vi "Main_12a.vi"() -> ()   [LabVIEW 2023]
uses:
  ENUM_Type.ctl
  <vilib>/Utility/error.llb/Trim Whitespace One-Sided.vi
panel:
  out "Complete Match Count":i32
  out "Answer":i32
  in  "Puzzle":string="??#.????#???.#?# 1,5,1,1,1\n?##?##??#? 7,1\n??????#???. 1,7\n??#?#??#.?#.??#? 5,1,1,2\n???????.??? 1,3\n?#..##?##??###??#? 2,13\n?.????????.???????? 1,5,1,6\n?.???#???. 2,2\n??#..#???#? 1,1,4\n?.?##?????#??? 1,5,2,1\n.???#?????##??#.? 3,8\n?????????????.#.. 4,3,1\n..#???????.? 4,3,1\n????#??.?.#??? 7,3\n#??#???##??.?? 4,1,3,2\n??#?#?##?.???#??. 6,5\n???.#??.??###?.#?? 3,1,5,2\n?.????##??#?? 6,3\n???..?##????.? 2,3,1\n?.?#????.??#?#.? 1,2,1,3,1\n?.?###.???? 4,2\n?#???..??##? 4,3\n???#????#?. 1,2,3\n#???#???#??#???.? 1,10,1\n???????????????????? 1,5,6,3\n???????#??? 2,6\n??.??.????.?#?????# 1,1,2,1,4,3\n???#???.??#? 1,4,1,1\n???#???##??##? 3,2,3\n????.??????#?.#? 1,1,1,4,2\n?.#??#???? 1,1,5\n??##???#?.##??..? 4,2,4\n??????#.????.# 4,2,1,1\n??????#??#?.??? 2,7,1\n.????????##.?.?.##? 5,2,1,1,2\n.??????????#?#. 3,1,2,1\n?????????????. 2,1,5\n?##????#?.?????.#??? 2,1,2,3,3\n?????????#?.?????#? 1,2,1,3,4,2\n..?.#???.?##.? 1,3,2\n.??????????????? 10,2\n?.?#????#?.??? 1,1,2,2\n??????.#??.?.? 1,1,1\n#???#?#??#????? 1,2,1,5\n???.?.??#????.? 3,6\n.#.???###???.#?..??? 1,8,2,2\n.???.??#????# 2,4,1\n.????#?#?? 3,3,1\n?###??#??## 4,2,2\n??#?#???#???.??. 3,5,1\n???####??##..?#.#.?? 9,2,1,1\n??#?#???#.?. 5,1\n???#????#???##?# 2,3,3,1\n?#???????#???#??? 1,3,3,3,1\n#???#????#.##..? 8,1,2\n?????.?#?#??? 1,5\n.??#.??#?.? 1,1,1\n?#?#???#???.??? 1,1,4,1,3\n.????#.?.#??? 1,1,2,1\n.??#?.??#? 4,2\n#????????. 1,4,1\n??.#?#????#?...?? 1,8,2\n?#.#?#.??##? 2,3,1,2\n...??.?#?? 1,1\n?.?.????#..? 1,2,1\n?##????????.??.?#??? 6,1,1,4\n?.??#.??.?.???? 3,2\n.????.?????.???.?? 4,1,1,3,1\n?????????##???????#? 2,1,1,2,2,2\n???.?????.????? 2,3,5\n???#??????.??#??.? 1,6,1,1,1\n??##??????###??? 12,1\n?.??.?????? 1,1,2\n??#??????#?.. 2,5\n???#####????. 1,8\n.?#?##??????#??.???? 6,2,1\n?.#??#???????#????? 1,1,12,1\n??????????#.?..?##? 1,1,1,1,3,3\n???????#???.??## 10,4\n.?#????.?.???..? 1,1,2\n.???#?#????? 2,2,1\n#????#?.????##?#?# 1,5,1,5,1\n???.##??????##??#? 1,2,8,2\n??#????????????#? 6,7\n????.??.#.?#?#? 1,1,1,1,4\n??##?#??.#???? 6,1,4\n?#?.?#????????#?. 3,2,4,3\n..??????##?# 2,1,2,1\n?????????.???? 4,1,1,1\n.??#?????.?.?. 1,6,1\n#.?#?#??????#??# 1,6,2,1,1\n.#?.#.##??# 1,1,5\n??#?????#?????? 5,4\n.#??.?.?.? 2,1\n.?#???##.????##?? 7,2\n?#?.??????#??????# 1,8,3\n?.#??#??.?#.. 4,1,1\n?#?#?#??????? 7,1,1\n?#???????? 6,1\n????#..?#???##? 1,1,2,3\n..?????#?###??.? 1,9,1\n?##???.???#?# 4,4\n??.??#???..??#? 1,2,1,3\n#?#??????.??#?? 8,1,3\n???#?##?#?? 2,6\n.?.???#???.#?????? 1,3,1,5,1\n?#.???????# 2,2,1\n?.???.??.? 1,1,1\n?#?#?#??????#??#??? 1,5,2,4,2\n?#??.?#?????.?#. 4,6,2\n#???.?#?#??#?.??#? 2,7,1\n.??#...???????. 3,1,1\n?..???##??. 1,6\n??#??#?#??? 2,4\n?.?.??.??????#?. 1,7\n?.?????????.??. 2,2,2\n???.?????? 2,1\n???.??????????? 1,3,4,1\n?#????#???#??? 10,1\n??#???.?????#???# 6,3,1\n????.?##??#??# 3,8\n?????????????. 1,7,1\n?..?????.#???.. 1,4,2\n?.???#???#? 1,5,1\n#???.????? 2,1,1\n?#.??#?.???? 1,1,1,1\n????.?#???.???. 1,1,4,2\n.?#??#??.??????? 2,4,6\n.??.?##.??#?#.??? 2,3,2,1,1\n..??????#?.?? 2,2\n???#?#??.##. 3,2,2\n?..?????????##?#??? 1,13,1\n??#?????#?.??#?????? 6,2,5,2\n???.???#???# 1,1,3,1\n??##????.?. 4,1\n??#??#??#?. 3,6\n.??????#????#.#.?? 1,1,8,1,1\n?#?#?.?.?.###??#???? 5,1,1,3,1,1\n???.#?#???.?? 1,1,5,1\n?????####??????? 2,5,2,1\n????.??#??#? 1,1,2,1\n??.?????#?#.????? 2,3,3\n?#??#?#?.????.??? 2,3,2,2\n?????????#??.??????. 1,6,1,1,1,1\n???.##?##??#? 1,6,1\n????#?.??.. 4,1\n?#??#?#???.????#?# 4,4,6\n?????#??#.#? 1,2,2,1\n?#?#?#??###??? 1,1,7\n.##?.????? 3,3\n??#???###????? 1,6\n.?###????????##?#?? 7,1,5\n..?#????????#? 3,5\n#?#???.??? 1,1,1\n#???????????#??.??? 10,3,1\n???##??#??#?.?????. 10,3\n?#?????.???????## 3,2,5,3\n??.??#####???. 2,8\n???.?????? 1,1,3\n???#???????????. 6,4\n#???#?????##???.?#? 2,1,1,5,2\n?#?..???#??????. 2,7,2\n?????##?#? 2,3,2\n.#?..????# 2,3\n???????#??#.?..??.. 3,1,1,2,1,1\n?.#??#????? 1,3,2\n???..?.?.? 1,1,1\n?#.?#??#???.##.? 1,1,4,2\n???#?#.??#??? 4,1\n??????#????.???? 6,1,1,1,2\n???..??.#???? 1,1,1,2\n????????.? 1,1,1\n?..#??.??. 3,1\n?##.??#??? 2,1,1\n?????#?????#?#?? 2,12\n?#??????#???.?? 1,6,2,1\n#??.???.??##???.#? 2,3,7,2\n???????..????#????? 2,1,1,7,1\n????#??.?????? 1,2,4\n?###?#?##?##??.??. 12,1\n?#??#.?.??#?... 3,1,1,1,2\n??#??#??#????#? 9,2\n???????##????? 1,1,5\n?.?#????#?.??.?? 3,3,1,1\n???..??????#..??#? 1,1,7,1,1\n??.???###???#..? 1,1,5,1,1\n??.??.#????#????# 2,1,7,2\n??????#?#??????# 1,6,1\n#?.?...??.??????? 1,1,1,6\n??#?##??#?..## 7,2\n?#?###..?.#?##??.?.# 5,6,1\n.??.?.???. 2,1,1\n?.???..?.?#?.??.???? 1,3\n.#?.??????.?.?#??? 2,6,4\n???##...??. 3,1\n????????????#?????. 4,6\n????#.??#? 1,1,1\n?.?#.??..??#?????..? 1,2,1,8\n?????.??.? 1,2,1\n??????##?.?? 1,4\n???.????#??? 1,1,5\n.??#???.#.#??#??. 6,1,2,1,1\n?.????#??##?????? 1,1,1,7\n??????##.??? 3,2,1\n?.????#?????.?.? 1,4,2,1\n?????????????## 1,1,2,4\n.?##??#??.??# 4,1,3\n??#?##??#?? 2,5,1\n?????.###??.?.#??# 1,1,4,1,1,1\n.????????##?#? 1,7\n??????????.? 7,1\n.?????###????..#. 12,1\n????.????? 3,1,1\n#.??#????#????#????? 1,5,1,7,1\n.##??????.??##? 7,3\n?..?.???#?????###? 1,1,5,5\n??????#???. 1,1,3\n??.#???????##????. 1,2,3,6\n?.?.?.?.#???????#?. 1,1,1,1,2,7\n?????#????????. 1,1,1,4,1\n?.??#??#?? 1,1,2\n??#???.#.?#?#?? 1,1,1,1,5\n?????????.? 4,1\n??.?????#?.?.#?? 7,1\n??.?#.?????#??. 2,7\n?????##..? 1,4\n?????????. 4,1\n??.?..?#???? 2,3,2\n????.####??###? 2,4,4\n?####???##??????? 10,1,1\n???#?#???# 1,5,1\n????###.??.?????#??. 6,1,6\n#???????#?. 2,1,4\n?#?.???##???????#? 3,1,2,1,6\n???#??#?.?.?????? 1,5,1,1,4\n?.#???##???.?.## 1,3,2,2\n???..##?.?.? 2,2,1\n?.#?#?????. 3,1\n????.##?#?#??##?? 3,12\n#?##???????? 1,3,3,1\n???.#?.????##? 1,2,1,4\n???.??#???? 1,3\n.???###??.???????# 7,5,1\n?#.??.?#???##?. 1,1,1,4\n.????###????? 2,6\n???#???.???????#?? 1,2,1,3,4,1\n.?.?????????? 3,5\n??#???#?.###????.?? 7,3,1,1,1\n#??###??#?#.????? 11,1\n#.?????#??#.##???.? 1,1,7,5\n??????.????#???? 1,1,4,1,1\n?.?#?#?#??###?? 7,4\n????#???#?#?###????? 1,2,10,1\n????#????? 1,4,2\n???.#??#????.?#??.?. 3,2,1,1,4,1\n?????.?#??????. 1,2,1,1,1\n?#???????#?#?#???.? 2,12\n?#??..??.???###?? 4,2,1,5\n##????????#.? 5,2\n#?#?.?.??###??#?. 4,8\n??##?.???? 3,4\n?.????##???????? 8,1,1\n#????#??#???#?#.??? 15,1\n?.?????.#? 4,2\n?.##???..?? 1,3,1\n#????#??????????#?? 2,7,2,3\n???.????#? 1,1,2\n??..#?????### 1,3\n????????.?? 2,4,1\n#??##??#.?????.??? 1,5,2,1,1,1\n???#.?#?#?. 3,1,2\n?##?#??????#?#.# 3,3,3,1,1\n??.#?..??? 1,1,1\n?#??.???#? 1,1,3\n???#???????.??##?? 8,3\n??.#.?#???#??.? 2,1,7\n??????.####?.?#?# 4,4,4\n??????????? 2,2,1\n?#?.??.???.? 2,2\n????#?#?## 6,2\n.??###??????.? 5,3\n.???#.#????? 3,5\n?##?#?.?#?#??. 6,2,1,1\n#.???.??#?####?..? 1,1,1,8,1\n????#???#???# 1,1,2,3\n?????.??.#???#? 3,5\n?#??..?????????#?. 1,1,3,1,4\n#?????????????.?? 6,1,1,1\n?#?????..?????#??# 3,1,1,5\n???????.???????????? 1,4,1,9\n.????????????.. 2,1,6\n.?#??????. 2,4\n??#??#???#.???#? 1,5,2,1,2\n.?.???????.?.#??? 4,1,2\n##?.??##?..???. 3,4,3\n??..??#??#?. 1,6\n??#??????????##???? 2,6,4,1\n??..????##?????? 1,5\n##????????.??.#??? 2,6,4\n?#??#...?????# 2,2,1,2\n?..??????.???.?# 1,1,3,1,1\n.?###??#???#???? 7,4,1\n?#?.?????. 2,2\n??..????.?????# 1,1,2,2\n??##.#??????.##??#?? 1,2,1,1,1,5\n??.##??????#???#??? 4,8\n??#?????????. 4,3,2\n#????.???? 1,1,1\n?..??.?????? 2,3\n??????#??###???? 1,1,9,1\n?????#?#???????.. 1,6,3\n?#??.???#?##. 3,3,2\n?..##?#???????#?? 9,1\n???.?#?#?#?. 1,5\n???##?#???#?# 8,3\n?##??#??.??.???????? 2,3,1,6\n.??...?????????#.#? 1,6,2,2\n????.#??#?#.##?. 1,1,1,3,3\n?#?#?????.??????. 5,3\n??.????##???. 1,5\n????#?.???? 2,1\n????..??#???. 4,2,1\n???????.?# 2,1\n????????????? 1,1,3\n???##??????###.?#? 2,2,2,3,1\n??????#?#?#?#?## 3,10\n?????#??..????????? 8,5\n??##???????.??? 6,1,1,2\n?.???.????.??? 3,1,1,3\n.?.???.??? 1,2\n.???###???#??.?? 5,1,1,1\n????#?.##?###.# 1,3,2,3,1\n.?#???????? 1,4\n?#?#?????????### 8,6\n?????..???.???? 4,3,1,1\n..?#?.?#??? 1,5\n.????.??#? 3,3\n?##????.?#??????..?? 7,3,3,1\n?????##??.?.??...?? 9,2,2\n??..#??####??.?.?#? 8,2\n??????##????? 1,1,6\n??????#??.???#? 7,5\n???#..??.????. 4,1,2\n.#?.?###??? 1,4\n????###?...?#?#? 8,4\n?????#???#??????? 1,1,6,1,1\n.??#?#?##??????? 7,1,1\n.#.?????#.?#### 1,2,1,1,5\n?#??..#??.#?? 3,1,1,1\n????#??.???. 3,1,3\n#.???#???. 1,2\n???.???##.???.? 1,1,2,2\n?#?#..?#????##?.?. 3,9\n.?.??.????? 2,2\n??????.?.##?#?.? 5,4\n???#???.????? 7,1\n??####?????.???#?? 6,3,4\n?.?...?#.#?#??? 1,2,5\n??.??#??#?#?#??.?? 2,3,7,1\n?#?.???????? 1,1,1\n????????#?##?#??? 1,2,9,1\n#???.???#????.??#??? 3,1,1,1,4,1\n.??#?.?.#??? 2,1,2,1\n.?##?###.###?#?.??. 6,5,2\n.?.???????#????##? 3,10\n?.##???..#? 5,2\n????????????#??.???? 1,1,10,1\n??##??#.??#??#?? 5,3,2,1\n?#???#.??????..# 6,4,1,1\n????????.? 1,2,2\n?????#??#??#????#??? 14,2,1\n???#??.???#?#???? 4,7,1\n.?.##?.???#??..????? 1,3,4,2\n??????#??????? 1,1\n..#?##??.????. 5,3\n??????????#.? 4,1\n#????.???.? 1,1\n.?..?#.??? 2,1\n?#.??##??.##?.?? 2,4,2,2\n??#????#??????? 9,1\n.#?.##?##.#???? 1,5,1,1\n?#?###???#??#?.??? 11,1,1\n???#??..?? 3,1\n#?#??????#?????#? 12,2\n??#?#?.???.? 2,2,3,1\n?#???.?.??#?#???? 5,1,8\n.???#?#??#?????. 10,1\n??????.?????.? 5,1,1,1\n.?.??????????# 3,7\n.#?.??..##??.?#..#? 1,1,4,2,1\n?##?#??.??###?????# 2,1,1,1,7,1\n?##?.???.? 2,1,1\n?????#.#?##.?#? 1,1,4,1\n?#?.??.?#.#.##.? 2,1,1,1,2\n???????.#.??##??.?. 6,1,3,1,1\n.?#??#???????#???.#. 3,1,1,2,4,1\n?????#?.##??##??.?? 1,2,2,3,2\n#??.???????? 1,1,1,1\n????#?.##?.?#?#?# 5,2,5\n.?.??.#?????????..?# 1,1,6,1,2\n???#?#?????. 7,2\n???????##??#?.?#?.? 1,8,3\n.?..?#?#???? 4,1\n??.?#??.????. 1,1,3\n????##???##???#??? 12,4\n?###?#??..#?.??? 6,1,2,1\n##??..##?#????# 3,2,1,1\n?????#?##??##???#?? 2,13\n#?..???##???##?#???? 2,6,4,1,1\n.????.?....#????. 1,3\n?.?.??#??#.?# 1,2,1,2\n???#??.??#.? 1,1,1,2\n.????#?#???#??????? 12,1,1\n?..#??#?##??#???? 1,1,2,3,5\n.#??##?##??????.?# 2,11,2\n.?.#?#?.?#???#.? 1,4,6\n?#.##??.????? 2,4,4\n???.??????.??. 2,1,1,2\n???????.?##.#???.? 1,1,1,2,3,1\n??..???????#?.? 5,2\n?????#????? 3,2,2\n.##????..#??.. 6,2\n????.??????.???###? 3,3,1,5\n??????#?.???# 1,3,1,1\n????#????. 6,1\n??.?#????. 1,4\n??????#???##???. 6,1,3,1\n?.?#.????. 1,1,4\n?##??.#?#??.#?? 3,1,1,1,1\n?.?#??????. 1,5,1\n???????#?. 1,4\n???#????#?##?#?????? 2,2,1,1,6,1\n??##.?????##??#.? 1,2,7,1\n????????.# 4,1\n.???#????? 1,1,1\n?.?#??.????.?#?? 1,4,2,2,1\n.?##?#???.??..?#? 3,3,3\n?#??.?.?#??? 1,1,4\n????..#????#.?? 1,1,1,3,2\n???#?..??? 5,1\n?##???##.?. 3,2,1\n??#???.???### 2,1,1,3\n????.?#??##?. 2,2,2\n?#???##??#?????#.??? 2,11,1\n???#??..?##??# 5,6\n????.??#???.#?#.?#?# 2,5,1,1,1,1\n?.??????#??? 2,3,2\n#.#???..????????. 1,1,2,6,1\n?.?..?.#??????##?? 1,1,1,1,3,5\n.??.?.???? 1,1,4\n#??#.?#?#???#??????# 1,1,2,1,1,8\n?????.?#..#. 3,1,1\n????##???.?????.. 5,3\n.????#???????? 1,5,1,1\n##?..#.???#?????? 3,1,1,2,1\n#??##???????????. 1,11,1\n????????#. 2,1,2\n.#?#?????????. 1,4,2,1\n#??#??.????????????. 5,5,2\n..?#?#???#???????.?. 9,1,1,1\n?#?.?????????... 1,6\n??###??#?#?.? 5,2,1,1\n.?????????.??... 6,1\n?.?.#??#??????#?#. 1,2,7\n??.?#?.#??.??. 1,2,2,2\n?##?#.?#?. 3,1,1\n??.??####???... 2,6\n.?????#????..?..??## 7,1,3\n.#?##???.? 5,1\n?.?.???#.???. 1,1,2,1\n?????.???## 1,3,2\n.????#??.??.?. 5,1\n.?#??.???? 2,4\n??#?.??#?? 2,2\n?.??.??????.?????? 1,1,2,1,1,5\n?????#??????.??? 1,5,2\n#..?#??.?# 1,2,1\n???????#???#?#???.? 5,8\n??.?#??#?? 1,2\n????#.#??#? 3,1,1\n#?#?..?..?????#??? 4,1,2\n??????.?##?##.??? 1,4,6,1\n?.????###??? 1,8\n??##???????##?????. 8,4,1\n?#.?#.?.?????? 1,1,1,6\n???#?.?.#??##???##? 2,10\n.?????#?.?##????#?# 1,3,2,5\n#?.?.?#?..???#? 2,1,1,2,2\n..???#??.??#?? 5,3\n.????##??? 7,1\n??#?###???# 7,1\n?????????????????. 10,5\n??#?#?????????###?? 3,1,1,1,4,1\n????##???.#??? 1,6,1,1\n.##??????##?..??#?## 11,2,2\n?#.????????? 2,1,1,2\n??????#?.??#??..???. 3,1,5,3\n.?##??????????#???? 3,1,1,1,2,1\n?#?...?#?????#?.? 2,8\n###?#.#?#?????.#???? 5,1,2,2,4\n?.???#?#.?????#?.? 6,5\n#????#???#???#?#? 2,2,3,3\n??#??.??#.?#? 2,1,1,2\n##.?...????????#?#? 2,9\n??#?#???#???? 4,1,1,1\n.???#?.?????.?#?.#. 4,1,1,1,1\n??#.?????#?????##? 1,1,1,7\n#???????#?????#? 1,1,8\n????##?#?#??##???#?. 1,8,6\n#.???.?????.#?? 1,1,2,3\n##?????#??.????#? 2,1,3,6\n#???###?##.? 1,4,2\n#..??????#???.. 1,10\n?????#???.?#?#??# 7,7\n???.#????#?????.#? 1,1,1,6,1,1\n??.#?#?????????.?# 1,4,2,2,1\n?#?#?..?#? 1,2,2\n?.?##.???###?? 3,5\n.?#????#??..?? 2,5\n???#.#??.?.????..#?? 2,3,4,1,1\n???#..?????.? 1,1,5,1\n?##?#??????##? 4,1,5\n??#.#?###?##?????#? 1,1,8,1,1\n.#?#??#.#?.? 1,1,1,1\n????????#?#?##??# 5,1,1,5\n.??#?.?#?????.?????? 3,7,4\n?#?????#.?#? 2,5,2\n????.?#????#?????#? 1,9,2\n?#????#???.??.??.. 7,2,2\n?#.##???????.?#.? 2,5,1,2,1\n?.##?#?.????#?#??. 2,1,6\n?###??#.#????##.?? 5,1,1,1,3,1\n.??#?????#???#?.# 3,1,2,2,1\n?.????.??.#?????? 1,3,1,5,1\n????##?##?? 6,3\n.?#???.?.????? 2,1,4\n?????...??.. 1,1\n??#????..??# 1,2,2,3\n?###.?????#.???#? 4,3,1,2\n???##????.?#.?#??? 1,2,2,2,5\n?#.?????.?###?##??.? 2,5,6,1,1\n.????.??.?????????? 3,10\n??.?#?#.#..??? 1,3,1,1\n?.?#?#??.?. 5,1\n???#.?????##???#??? 2,13\n??#???#.#???#???#?? 2,2,11\n?#???????? 4,1\n??????##???##????# 2,10,1\n???#????#?? 3,1\n##????#.?.? 3,2\n.????#?????? 6,1\n?.??.????#? 1,4\n?????????.? 1,4\n#?#??#?##????#????#? 14,3\n#..#????#??? 1,1,4,1\n.?.##????.?? 1,2,1,2\n???.#??#?#?.?????? 1,1,7,1,1,1\n..?#????.#???##????? 3,2,7\n?????.??.? 3,1\n.?#??#?#..?#?.?##.?? 2,4,2,3,1\n???#?????.# 8,1\n????..##?.??#? 1,2,3\n.?????.?#? 1,1,1\n??#?.#?#?#?.###?. 1,5,4\n???.#????##.???##? 1,3,3,5\n?????????#?#?????? 7,2,1,1,1\n#.?##.???.?#?..?.#. 1,2,1,2,1,1\n???#.???.?? 1,1,3\n??.?.??###??.????.? 1,1,7,1,1,1\n.?.#.?#?##?.???# 1,1,5,1,1\n???###?#???# 8,2\n?.????.#..##??? 1,1,2,1,4\n??#????####???#?. 3,8\n#..?#????##?#?. 1,3,3,2\n###.??.##.? 3,1,2\n???##?.????#?#??? 4,5\n?.??.?.?.??? 1,1,1,1\n.#???##??#???##???? 1,1,5,4,1,1\n?..##..??#...?.?.?? 2,1\n?#..#???.?.??# 2,2,1,1\n????#?.#??.? 1,3,1,1\n?#?????#???.????? 3,3,1,2\n#.????###???.?#???? 1,7,2,2,2\n?????.?????? 3,1\n.??#???????. 3,1\n?.?#??.?#???##?#?? 1,1,1,11\n?#????#?#. 4,1,1\n..#?###???#.??? 1,7,2\n#....????? 1,1,1\n?.????????.? 4,1\n##?.??????.#??? 3,2,1,1,1\n?????.?#.?????#??.. 2,3\n?#??##?#?#?.??##? 7,2,3\n.?.?????##.??? 1,2\n.#?##?##?.?????.?#.. 7,1,1,2\n???..???#?. 1,1,2\n...?.???#?#? 1,4\n?????#????#.? 7,2\n??#????##???##. 3,2,4\n???.???????. 2,1,1,1\n###?..?????.. 3,4\n.???????????..?. 4,2,1\n?.?.#??.?? 1,1,1\n?????????????#?? 6,6\n..#?????.??? 4,1\n???#??#?##.?#?.?? 7,3\n#???###??????#?? 1,1,3,2,3\n?##??.??#??????#???# 3,9,1\n???#??#??.??????#??? 7,3,1\n.???###??##?#.?.??? 6,2,1,2\n?.?#?#?.?.?#? 3,2\n.??#.?###???##?? 2,5,3\n????.?????#??###?? 3,12\n?#?##?#..#??#?? 5,1,1,2\n??#??...???#?#???. 1,7\n???##???.???#.?. 7,3\n??.#???#.# 1,5,1\n??###???????????# 5,4,3\n#??..#??##.?????.? 1,1,5,2,1,1\n????#.???#????.. 3,4\n#?????.#??? 3,2,3\n?#?.???????. 2,2,2\n?.?????????## 1,1,4,3\n#????????..#?#????? 3,1,1,3,4\n???#??#??????????.. 7,1,1,2\n?##.??###???#?#??# 2,1,3,1,3,1\n?#?.???#?#?#?.??# 3,5,2\n??#????.??#?#? 3,3,4\n###?##???#?#??.?.# 8,3,1,1\n.??.?#???#??? 2,1,3\n.???#??###?? 1,6\n???????.???????? 7,1,2,1\n.??###?.??#.? 5,3\n?#???#???????#?#???? 2,5,1,4,2\n????.?????#?????? 1,1,7\n.??.?.?#?##?#???#?? 1,11\n?????#???? 5,2\n?.??.???.#?? 1,1,3\n????#???????? 5,3,1\n#?##????#???#?.?#.# 4,3,1,1,1\n??#??????#?? 1,1,1,4\n.????.#?????#?? 1,2,1,1,3\n????????????????? 1,4,3,2\n????.#?.##?##?#?#?? 3,1,5,3\n??#?###??? 1,3,1\n????#???....? 8,1\n.????.???.???..???. 2,3\n?????.??#? 4,2\n#??.#.????#.???###? 2,1,1,1,1,4\n.???????.??????# 6,5,1\n??#??#?????.??#. 1,4,1,2\n??#?.??.??????#?#??? 4,1,3,1,5\n?#??#???????#..??? 4,7,1\n???#?##?????.?? 5,2,1\n.?###?????#?##??. 6,7\n#??#..??????#?? 1,1,7\n.??#?#??????# 4,1,2\n.###??####????#???# 4,13\n????#?????.?. 6,1\n#?##???#????? 5,1,2\n??#?.##??????????? 4,4,5,1\n.????#???? 2,1,3\n?.?#.???????#?.????. 2,4,1,1,3\n?.?#?????##??????? 2,10,2\n?????..???##? 2,3\n?#.#.???#???.? 1,1,1,4\n.?##???##?????###??? 15,2\n?#.#?.????.??.?#?.? 1,2,3,1,1,1\n????#??????. 5,1\n?.#.????##??.?. 1,7\n??.?#?..??#?????.? 2,6\n???##?.#?.?#? 3,2,2\n?#?.???.?? 1,2\n?????????..?#??? 1,1,2,2,1\n?#.??..??? 1,1,2\n??.????##???? 1,1,3,1\n??####??????#.?.??? 5,1,1,1,1,1\n.??#????.?# 2,1,2\n..#?#???##???.?.??# 1,1,4,1,3\n??.##..??. 1,2,2\n?#???#?????? 2,5\n????##?#?.???.? 5,1\n.?#?..????#??.??? 1,4,1\n.#####??????#??. 7,5\n???.?.?.##?#???. 1,5\n????###??.????#?? 8,5\n?????#.???#?.?.?# 4,4,1,1\n????????.?###????#? 1,3,4,1,3\n?.?????.?#?????# 1,3,1,2,1\n??.??????????? 1,3,1,1\n???.?????#??? 1,6\n?##???#?#????#????#. 3,3,3,2\n??#?.?.???### 2,1,3\n#??..?##??????.??? 1,1,3,1,1,1\n???#??.?.#???#? 6,1,2\n?#?..????? 3,2\n?##??#???? 5,2\n??.??????.?#? 1,4,2\n.#?##???.???#??????? 7,4,1\n?.#???..????? 4,3\n.???..?#??##?? 1,7\n.#???????.??? 1,1,1,2\n?#?#???????##. 6,3\n#.?.#?????#??#?#???. 1,1,1,6,4,1\n.???????.?#?#??????? 2,5\n??.?.?????? 2,3\n???.????..#? 1,1,1,2\n??#??.?#?..???##??## 2,3,8\n#??.?.?#??#?. 2,5\n?.????.????????? 1,2,3,1,1\n???.??.??????????#. 1,1,1,3,3\n???????.??? 1,1\n##??#????????.?????# 2,2,6,1,3\n??.?????##????## 2,1,1,8\n???.??#?????#??.. 1,3,6\n??#?#??#???????.? 7,1\n.?#.????#??#? 2,4,2\n?????.??#.??? 1,2,2,1\n??##???.????????. 6,6\n..???..?.?.? 3,1\n??#?.??????.. 2,1\n???????##?????. 1,1,4,2,1\n??##..??#???. 2,4\n?????#??????#? 1,2,4\n..??#???#?????#?? 3,2,5\n???.??#??.???#?#??? 2,5,6,1\n?#?#.??##.?. 3,3\n#??#.?????.?? 4,2,1\n?#???.?#???#???.. 4,9\n????.??????#?#??# 2,7\n??#.??????????????? 3,7,5\n??#????###? 1,4\n???#????#.#.??.. 1,3,2,1,1\n???#?.???? 1,2\n?.??.?#??? 1,3\n??.????#??#.?.? 1,2,1,1,1\n..??????.?? 4,1\n??#?.???.???? 3,1,1,2\n?.????#????#? 4,3\n?#?????????????? 5,4,1,1\n?..?????#? 1,1,1\n?.?#???.?? 4,1\n#??#.????? 4,4\n#??.?????????????? 2,1,1,3,2,2\n.???#????.?? 1,1,2,1\n??.?##?.??#??#?#??.. 4,10\n????##????#???#.???? 2,3,2,1,1,1\n????????.??###?????? 7,5,2\n????.?.#??? 2,1,1\n.#?..?#????#???## 1,12\n#???##??.???????? 1,5,2,1,3\n???#???#?.#??..? 7,1\n?#????.???.?#? 6,2,1\n.#?????????#???. 6,1,3\n???###????????#?#?#? 8,2,1,4\n?#?#..??#???. 4,1,3\n.???##?#.??? 1,4,1\n??????????? 5,1,1\n??.#?#.???? 1,3,3\n.#.###??????.#? 1,4,1,1,1\n???#??.?.????? 1,3,4\n?#.#????????????# 1,1,1,8,1\n.??????###? 3,3\n.#???????#???? 3,1,4,1\n??#??.?#???#...? 3,6\n?#???????.?#???.???? 9,4,1,2\n???#.??#??? 4,3\n??#????#?#.??.?# 1,3,4,2\n????#?##?.??????? 6,1,2\n.??##?#?###..#??.?? 3,5,2\n??###???##?#?.??. 12,1\n?..#?????#????#?# 2,1,2,4\n????###?.?#??#??#. 8,6,1\n????##?#????# 10,1\n#?##?..?##?? 5,3\n?#.?#??#???????? 1,7,2,2\n.#?..?#?#??#. 2,6\n#??#????.??#?#. 7,3,1\n.?.??.????. 1,1,3\n?????.???#?#??.?? 1,3,4,1,2\n????????????#??#?? 4,8\n????####?#? 1,7\n?.#????.????#?.?? 1,6\n?#?????#?##?? 3,4\n?#????#????# 9,1\n?##?#?????.??? 6,1,1,1\n???..?##?..?????? 2,2,3\n#.??.??????? 1,1,2,1\n?##???##.?###? 3,2,4\n#?##????#.? 6,1,1\n.????.??###???#? 1,2,5,2\n?.#??.??#???? 1,3,4\n??##????#???#?#??? 4,7\n?#?.???#??##???#?? 1,1,2,8\n???.?#?##????.? 1,7\n#.?##?#?.#.????# 1,5,1,1,3\n#???..??#????#????? 4,5,2,1,1\n???????.???????#? 1,3,1,2,1\n##???????? 3,1\n?#..?.???? 1,1,1\n..??.#???##???#. 1,10\n.?????##?????#????. 7,4,1\n??..#?..#.#.#?. 1,2,1,1,2\n????.?###?#??. 2,8\n????.#?????? 3,6\n??#??#????#.?.?#.??. 10,2,2\n???#??????????? 8,2\n???.????#??..?. 1,5\n.?.??..?#. 1,1,1\n#??###..???#???? 6,1,1\n???###?..#?#??????? 5,7,1\n????#??#??#?#?.??#? 1,1,2,5,3\n????#??.?.?#???#. 7,1,1,1,1\n?##?#?#?.??#?. 6,1\n???????#?#???.# 1,4,1,1,1\n???????##.?# 9,1\n.?????#.???. 1,2,1,2\n#.?#.??#?? 1,1,1\n?##?#?????? 5,4\n?.?##??.#? 4,1\n?????##???.#?.##? 1,5,1,2\n??????.??? 1,1,2\n?.??.?#?#?#.?##??#?? 6,8\n??#???????????.?? 8,1\n#????????###??#??#? 1,2,8,1,2\n#.#???#?#?#.?????#? 1,9,1,1,1\n#.??#???##? 1,7\n?????##?????????#??? 6,1,2,4\n????#?##??????#?#?# 2,4,3,3\n?#?.##????#???? 1,3,2,1\n?.?.??#?.? 1,1,1\n???????#?#???..??? 1,4\n???.?#??##?#?##.#? 2,10,2\n??#?#???..???.??.? 7,1,1\n?????????.#.??????.? 6,2,1,1,3,1\n?#???##????# 2,6,1\n#?###?#??.#??..#.? 7,1,3,1,1\n???.???#???#?? 1,5,1\n??????#??????.???#? 7,4\n#?????#??.???#.? 3,3,1,1\n?.?..??.?##????.? 1,1,3,3\n?##????.???? 7,1,1\n?.?##.?#?#?????? 3,3,2\n?.??.?.??? 2,3\n?##?..????? 3,5\n??####?..?? 4,2\n???.???????????????. 1,7,6\n#???####???.# 8,1,1\n.#.???#?.????.? 1,2,3\n????????????#?????? 2,3,9,1\n#?#??#????????? 1,5,1,1,1\n.?.????.?#.?. 2,1\n????..#??? 1,1,1\n??##?????#???? 4,7\n?##?????.?#? 5,2\n???????###????##?# 3,1,6,2,1\n##?????.???. 4,2,2\n??#??.??#?..# 1,3,1\n????.#???????#?.. 1,10\n####??###????#.???. 5,3,3,3\n?#.?#???.?#? 1,4,3\n#.?#?#???#.#??????? 1,4,2,1,1,1\n??#????#?###???#?# 5,11\n??.???#???#????????? 1,5,3,1,2\n.??????#???####?.#?? 13,3\n.??????#?#?.??.?#? 10,1,2\n??..??##?#??????.??? 10,3\n????#???#####?????.. 10,2\n????#?#??#???###? 3,7\n????.#?.?????#.? 1,2,6\n???????????..? 1,4\n?.???#?????.? 1,2,1,1\n#??#??#?#???#?#.?? 1,8,3,2\n?????###????.???? 1,5,3\n???###?#?##????.??.? 1,9,1,1\n.?#?##???#????##??.. 9,3\n.?.?.?#????????##?. 1,1,1,1,1,4\n?.??.??#????##??##?? 3,6\n??????#?????.#?? 6,1,3\n?#?#???????.?#?.???. 11,3,1,1\n?.?#..#??????.??. 1,1,6,1\n??????#???### 3,8\n???#?#??.??##????#?? 8,1,8\n.#?.??.??#? 1,3\n?????.??????#?????. 2,1,1,10\n??.#????#.? 1,2,1\n???#?????????#?#?? 4,8\n..??..?????.### 1,2,3\n??.???#???.??# 1,7,1,1\n?###??..?.??#??#???? 5,4\n????????#?..?? 2,5,1\n???##?#?????#### 2,2,1,7\n?????#???#? 5,1,1\n??#.?#???####??#??.? 1,11,1\n?#?????##?#?? 5,5\n??.??.?####?. 1,6\n.???????#?????. 1,6,1\n????#.?????.??.?#? 1,1,1,2,1,2\n???.?#?????#.?#?.??? 1,4,1,1,2,3\n.#??????.#?? 1,1,1,1\n..#?.??????????? 2,5\n.??##???????. 3,4\n??#????#??????????.. 1,4,9\n.??#??.#.?# 2,1,1\n??.??????.?#????? 1,4\n#.?#??#???##? 1,2,7\n?###??.#.??. 4,1,1\n???#???#???. 7,1\n?????????#??? 4,4\n???.???????#.? 1,3,2\n?#??????##? 4,1,3\n?#.??.??#?.# 2,2,2,1\n?.#?????.????? 2,1,5\n?.#???#.?#?## 1,1,2,5\n#?#.?##???????#??.# 3,3,1,2,1\n#?#???.?.#.#??# 5,1,1,1,2\n??##?.##?????? 2,7\n.??###?#??#???? 5,1,6\n?.???#?????.?#??? 1,6,2\n??.?.?#??.???.???? 1,1,1,1,3,1\n???.???.###?##???## 1,1,1,6,3\n#???#??##??# 6,2,1\n??##??.##????? 3,7\n?#?#?#?.???##???.?#? 4,1,7,2\n.??#?#????.?##.? 8,2\n.???#???.. 1,1,1\n.????#??.#?#?. 2,4\n#?.?????????..?? 1,1,1,4,1\n?#???#??.? 1,2,1\n#???????????.???.? 4,3,1,1\n????#?#???#???#.?. 12,1\n???.??#.?#???#? 2,1,7\n??#?.#??.?#?. 1,1,2,1\n??#.???#.?? 2,2\n?????#??.????? 7,4\n?#?????????###?????. 1,1,1,1,5,2\n.?#?.#???? 2,3\n???###?#?..??.#?# 2,6,1,1,1\n..#?.???#?#???#??? 1,12\n????##.???? 3,2\n?#?????##?????? 1,2,5,1\n??????#???# 3,1,3\n.##??.???.? 3,1\n???##????...??..??? 6,2\n???????#???. 1,4,1\n?#??#???##?.??.# 10,2,1\n?.?.???#??? 1,1,3\n?#?#?#??..?? 8,1\n??#?.???????#?? 1,10\n?.#???#?#??????? 1,2,4,1,3\n#?#?.?##?????. 4,6\n#?#??.???#? 3,4\n?.?????#?#??. 1,8\n?.?.?.#.??.??#? 1,1,1,1,3\n?#???##??????##???.? 9,4,1\n?#???????????.? 5,1,1\n#???.??#?#????#?#? 2,1,11\n??#???????#???????? 6,1,7,1\n?#???#???????#?. 1,4,1,2\n????#??.???#.?? 6,2,1,1\n???.?#????.# 2,2,1,1\n#???#..??#?#????.? 5,7\n##?#..???.??.#?# 4,1,1,3\n.?..???????.????.?.. 2,3\n.???????.?? 4,1,1\n.?####??#?? 4,1\n??????#????#???? 1,1,6,3\n??#???#.????#??. 6,2,4\n?????????.#?? 5,2,2\n??#??..??????? 3,3\n.#?.??????#???. 1,2,1,1,1\n????????.?#????? 1,1,1,2,2\n?.??.??#??#?? 1,5\n.???#??????# 1,1,5\n?#?????.#?#?????? 2,1,1,3,5\n???#????#????#??#?## 1,1,4,2,5\n?.??.#.????..? 1,3\n??????#?#??? 8,1\n??#??.????#??.? 3,5\n?????#.?????#?#???.. 2,2,6\n????#.???. 1,1,1\n???#?.???#????# 1,2,9\n??#?#???###????#? 1,3,1,8\n#.???##??##? 1,1,2,2\n????#?????.#?.. 5,2\n..????.?????? 3,4\n????.??????? 2,1,2\n.?#??????????.? 7,2\n???#??????#?? 2,2,4,1\n???##?????#??#?. 1,9,2\n#????????.#??.? 1,3,1,1,1\n.??.#???#?##??.?? 1,2,2,4,2\n???.?????#. 1,2,2\n????#????.??? 5,1,1\n.????.??#?#?#???.? 3,5,3,1\n??????##??#.??? 1,2,5,1\n??????##.??.????.? 8,2,1\n?.?.?.?#?#?.????#?. 4,6\n..?????.?#??? 1,1,5\n???#?????????# 1,6,4"
  in  "Example":string="???.### 1,1,3\n.??..??...?##. 1,1,3\n?#?#?#?#?#?#?#? 1,3,1,6\n????.#...#... 4,1,1\n????.######..#####. 1,6,5\n?###???????? 3,2,1"
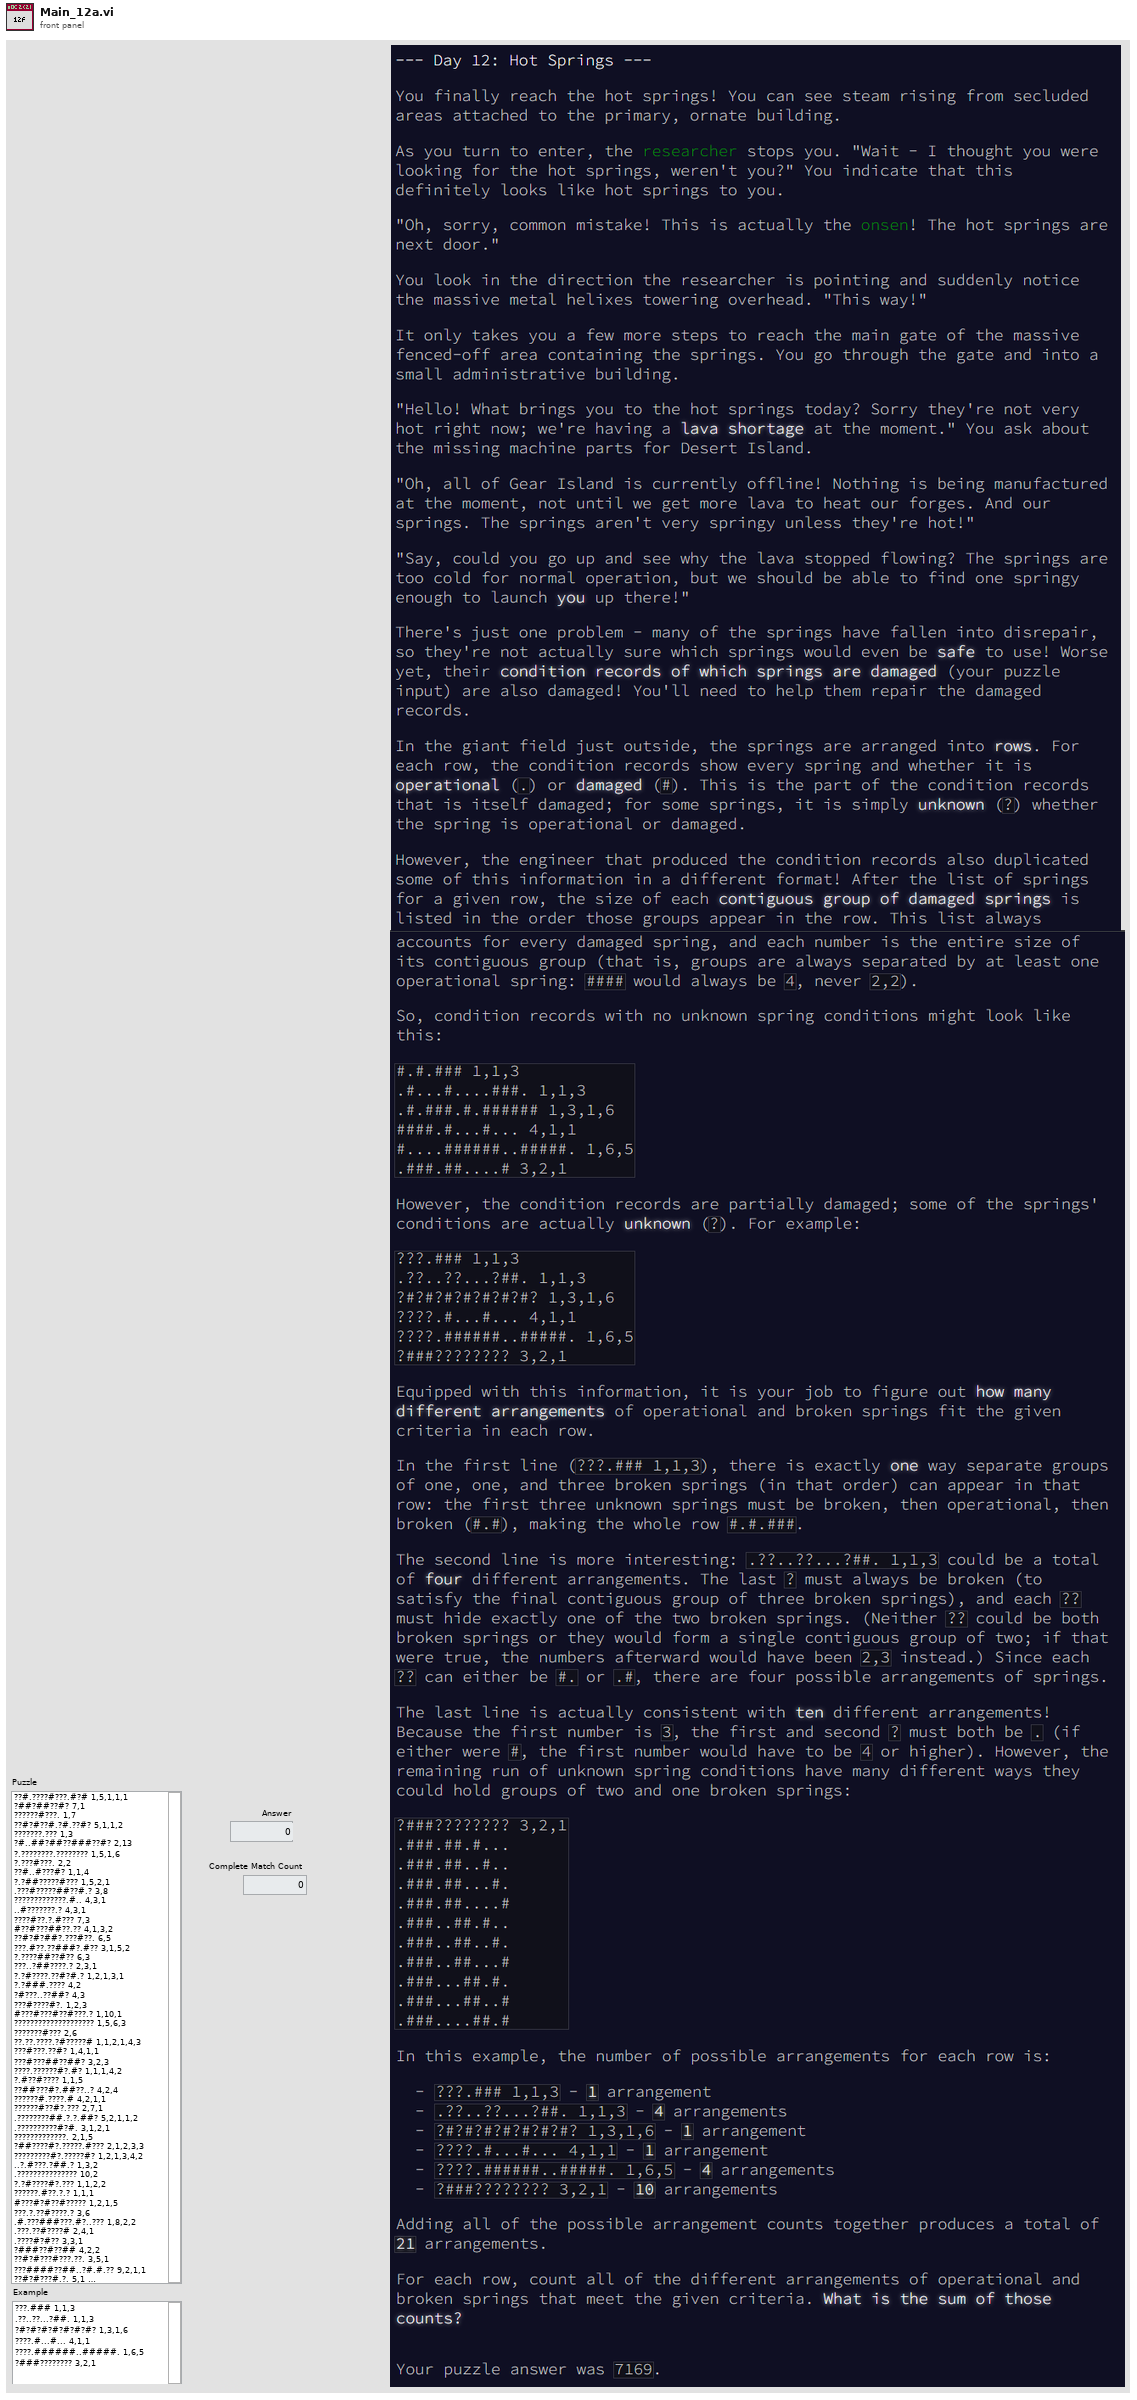
[diagram p1: front panel]
types:
  T1 = typedef "ENUM_Type.ctl" = enum16{"Damaged", "Operational", "Unknown"}
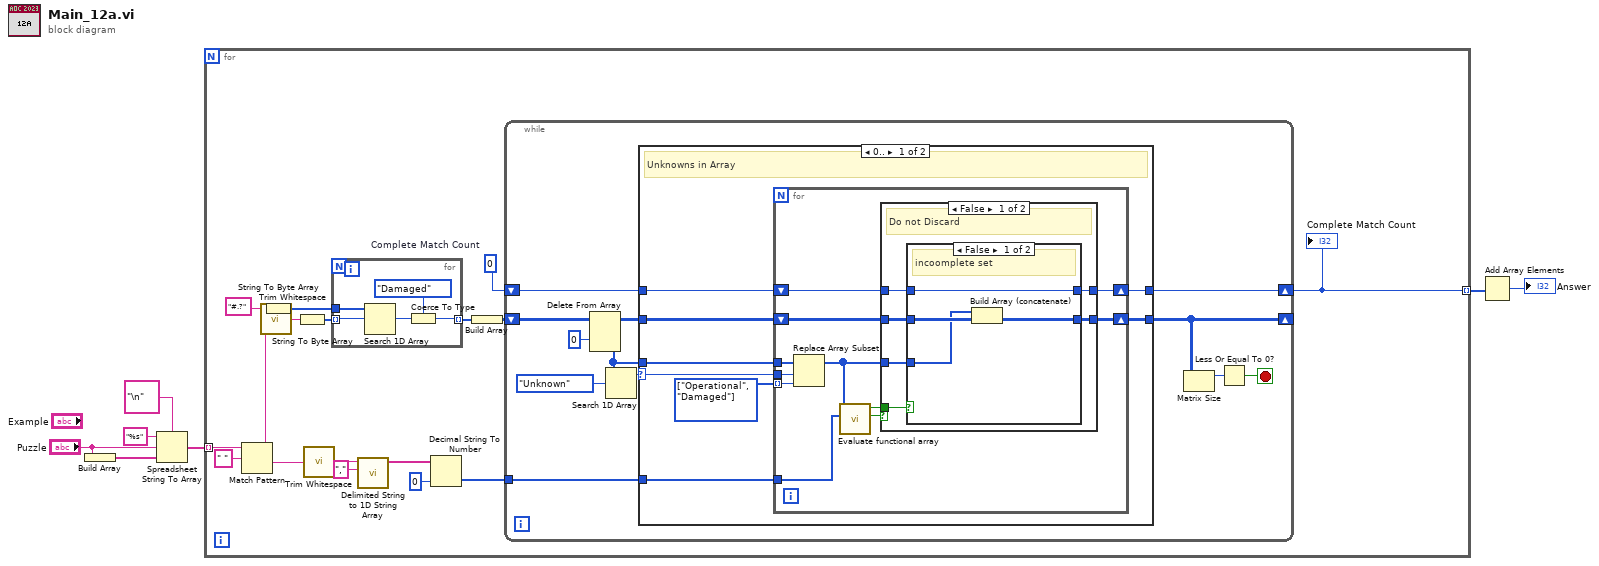
[diagram p0: block diagram]
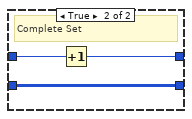
[diagram p2: hidden frame]
diagram:
  n1 = Build Array("Puzzle") -> (w7:string[])
  n2 = Spreadsheet String To Array(delimiter (Tab)="\n", format string="%s", spreadsheet string="Puzzle", array type (2D Dbl)=w7) -> (array=w4:string[])
  n3 = for {
    tunnel: w4 -> [w24] mode=indexing
    tunnel: [w8] -> w2 mode=indexing
    w9 = 0  # Complete Match Count
    n4 = Match Pattern(string=w24, regular expression=" ") -> (before substring=w18:string, after substring=w19:string)  [unwired: 1 in, 2 out]
    n5 = call <vilib>:"Trim Whitespace.vi"("string"=w18) -> ("trimmed string"=w17:string)  [unwired: 1 in]
    n6 = String To Byte Array(string="#.?") -> (unsigned byte array=w20:u8[])
    n7 = String To Byte Array(string=w17) -> (unsigned byte array=w22:u8[])
    n8 = call <vilib>:"Trim Whitespace.vi"("string"=w19) -> ("trimmed string"=w16:string)  [unwired: 1 in]
    n9 = for {
      tunnel: w22 -> [w76] mode=indexing
      tunnel: w20 -> [w77]
      tunnel: [w73] -> w11 mode=indexing
      n10 = Search 1D Array(1D array=w77, element=w76) -> (index of element=w75:i32)  [unwired: 1 in]
      n11 = Coerce To Type(0:w75, 1:ENUM_Type."Damaged" ("Enum")) -> (2:w73:T1)
    }
    n12 = call <vilib>:"Delimited String to 1D String Array.vi"("delimiter"=",", "delimited string"=w16) -> ("string array"=w14:string[])  [unwired: 9 in]
    n13 = Decimal String To Number(string=w14, default (0L)=0 ("default (0 I32)")) -> (number=w12:i32[])  [unwired: 1 in, 1 out]
    n14 = Build Array(w11) -> (w10:T1[][])
    n15 = while {
      shift-right: [w35] -> _
      shift-left: w10 -> [w32]
      tunnel: w12 -> [w27]
      shift-right: [w25] -> w8
      shift-left: w9 -> [w26]
      stop <- w33 stop-if-true
      n16 = Delete From Array(array=w32, index (row)=0) -> (deleted portion=w28:T1[], array with subset deleted=w31:T1[][])  [unwired: 2 in]
      n17 = Search 1D Array(1D array=w28, element=ENUM_Type."Unknown") -> (index of element=w29:i32)  [unwired: 1 in]
      n18 = case shown="0.." w29 {
        selector: w29 -> [w42 _]
        tunnel: w31 -> [w41 w72]
        tunnel: [w40 w72] -> w35
        tunnel: w28 -> [w44 _]
        tunnel: w27 -> [w43 _]
        tunnel: w26 -> [w39 w71]
        tunnel: [w38 w71] -> w25
        frame 0.. {
          w37 = T1[] [enum."Operational", enum."Damaged"] items=["Damaged", "Operational", "Unknown"] ("new element/subarray")
          # "Unknowns in Array"
          n19 = for {
            tunnel: w44 -> [w55]
            tunnel: w43 -> [w54]
            tunnel: w37 -> [w53] mode=indexing
            tunnel: w42 -> [w52]
            shift-right: [w49] -> w40
            shift-left: w41 -> [w50]
            shift-right: [w46] -> w38
            shift-left: w39 -> [w47]
            n20 = Replace Array Subset(array=w55, new element=w53, index=w52) -> (w45:T1[])
            n21 = call "Evaluate functional array.vi"("Number Array"=w54, "Function Array"=w45) -> ("Discard"=w51:bool, "Complete Set"=w48:bool)  [unwired: 8 in]
            n22 = case shown="False" w51 {
              tunnel: w50 -> [w60 w70]
              tunnel: [w57 w70] -> w49
              tunnel: w48 -> [w61 _]
              tunnel: w47 -> [w59 w69]
              tunnel: [w58 w69] -> w46
              tunnel: w45 -> [w56 _]
              frame False {
                # "Do not Discard"
                n23 = case shown="False" w61 {
                  tunnel: w60 -> [w64 w66]
                  tunnel: w59 -> [w65 w68]
                  tunnel: [w65 w67] -> w58
                  tunnel: [w63 w66] -> w57
                  tunnel: w56 -> [w62 _]
                  frame False {
                    # "incoomplete set"
                    n24 = Build Array (concatenate)(w62, w64) -> (w63:T1[][])
                  }
                  frame True {
                    # "Complete Set"
                    n25 = Increment(x=w68) -> (x+1=w67:i32)
                  }
                }
              }
              frame True {
                # "Discard"
              }
            }
          }
        }
        frame ..-1 {
          # "Complete Array"
        }
      }
      n26 = Matrix Size(0:w35) -> (1:w34:i32)  [unwired: 1 out]
      n27 = Less Or Equal To 0?(x=w34) -> (x <= 0?=w33:bool)
    }
    "Complete Match Count" <- w8
  }
  n28 = Add Array Elements(numeric array=w2) -> (sum=→"Answer":i32)
